vi "Go To Height.vi"(6 "Synchronization":enum16{"Start", "Wait"}(ring), 7 "Description":string, 8 "Command Info In":T1, 11 "Height":dbl) -> (0 "Command Info Out":T1)   [LabVIEW 2018]
doc: "This template has a parameter to control whether it waits for the command to complete or not. This is useful for operations that have a timed duration or a sensor-based duration. \n\nBe sure to right-click and select New from Template and save with a new command name."
uses:
  <vilib>/Rock Robotics/WPI/Framework/Command Status Info.ctl
  <vilib>/Rock Robotics/WPI/Framework/Completion Status.ctl
  <vilib>/Rock Robotics/WPI/Framework/Completion Notifier.ctl
  Implementation/Arm Setpoints.ctl
  Implementation/Arm Operations.ctl
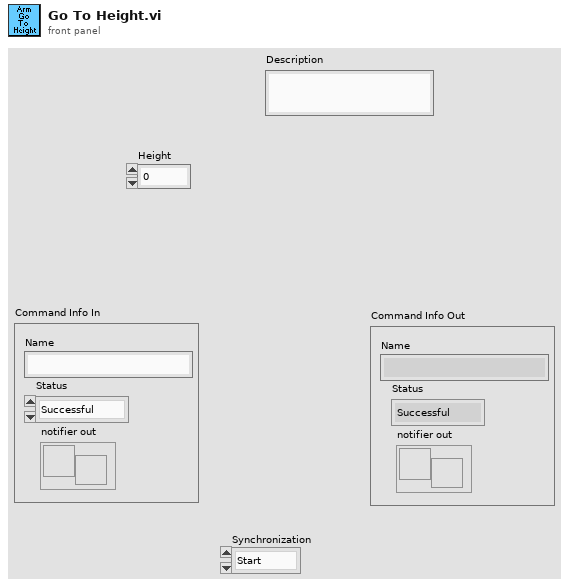
[diagram p1: front panel]
types:
  T1 = typedef "Command Status Info.ctl" = cluster{"Name":string, "Status":T2, "notifier out":T3}
  T2 = typedef "Completion Status.ctl" = enum16{"Successful", "Aborted", "Incomplete"}
  T3 = typedef "Completion Notifier.ctl" = refnum<notifier>
  T4 = typedef "Arm Setpoints.ctl" = cluster{"Operation":T5, "Speed":dbl, "Time":dbl, "Height":dbl, "DistanceForDrive":dbl}
  T5 = typedef "Arm Operations.ctl" = enum16{"Reserve", "Read Current", "Immediate", "RaiseForTime", "GoToHeight", "StayAtHeight", "RaiseAfterTime", "RaiseAfterDriveAtDistance"}
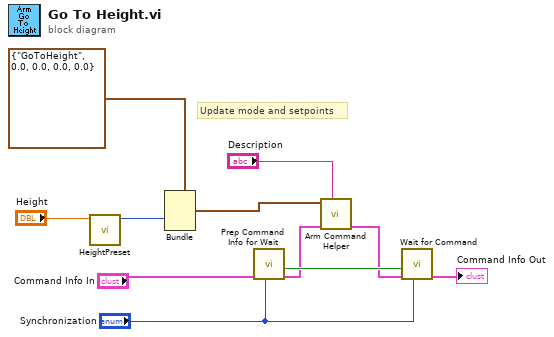
[diagram p0: block diagram]
diagram:
  # "Update mode and setpoints"
  n1 = call "HeightPreset.vi"("Height"="Height") -> ("Sensor Units"=w2:i32)  [unwired: 10 in]
  n2 = Bundle(cluster=T4 {"Operation"=enum."GoToHeight", "Speed"=0.0, "Time"=0.0, "Height"=0.0, "DistanceForDrive"=0.0} ("SubSystem Data"), "Height"=w2) -> (w4:T4)  [unwired: 4 in]
  n3 = call <vilib>:"Prep Command Info for Wait.vi"("Synchronication"="Synchronization", "Command Info"="Command Info In") -> ("Command Info"=w8:T1, "Allocated"=w9:bool)  [unwired: 8 in]
  n4 = call "Arm Command Helper.vi"("Description"="Description", "Command Info In"=w8, "SubSystem Data"=w4) -> ("Command Info Out"=w5:T1)  [unwired: 6 in, 2 out]
  n5 = call <vilib>:"Wait for Command.vi"("Synchronication"="Synchronization", "Command Info in"=w5, "Allocated"=w9) -> ("Command Info out"=→"Command Info Out":T1)  [unwired: 8 in]
